vi "canDataSort.vi"() -> ()   [LabVIEW 2023]
panel:
  in  "canArrayDataIn":string[](array[string])
  in  "canArrayID_In":string[](array[string])
  in  "e":string="         2  1FFFFFFF   00000004    8        00\t00\tFF\tFF\tFF\tFF\tFF\tFF\r\n         3  0CF101A7   00000004    8        68\t00\t97\tCC\t00\t15\t39\t1A\r\n         2  1FFFFFFF   00000004    8        00\t00\tFF\tFF\tFF\tFF\tFF\tFF\r\n         3  0CF102A7   00000004    8        30\t75\tE0\t2E\t80\tFF\tFF\tFD\r\n         3  0CF101A7   00000004    8        68\t00\t97\tCC\t00\t15\t39\t1A\r\n         2  1FFFFFFF   00000004    8        00\t00\tFF\tFF\tFF\tFF\tFF\tFF\r\n        12  1FFFFFFF   00000004    8        00\t20\tFF\tFF\tFF\tFF\tFF\tFF\r\n         3  0CF102A7   00000004    8        30\t75\tE0\t2E\t80\tFF\tFF\tFD\r\n         3  0CF101A7   00000004    8        68\t00\t97\tCC\t00\t15\t39\t1A\r\n         2  1FFFFFFF   00000004    8        00\t00\tFF\tFF\tFF\tFF\tFF\tFF\r\n        22  1FFFFFFF   00000004    8        00\t20\tFF\tFF\tFF\tFF\tFF\tFF\r\n        12  1FFFFFFF   00000004    8        00\t20\tFF\tFF\tFF\tFF\tFF\tFF\r\n         3  0CF102A7   00000004    8        30\t75\tE0\t2E\t80\tFF\tFF\tFD\r\n         3  0CF101A7   00000004    8        68\t00\t97\tCC\t00\t15\t39\t1A\r\n         2  1FFFFFFF   00000004    8        00\t00\tFF\tFF\tFF\tFF\tFF\tFF\r\n        23  0CF101A7   00000004    8        68\t00\t97\tCC\t00\t15\t39\t1B\r\n        22  1FFFFFFF   00000004    8        00\t20\tFF\tFF\tFF\tFF\tFF\tFF\r\n        12  1FFFFFFF   00000004    8        00\t20\tFF\tFF\tFF\tFF\tFF\tFF\r\n         3  0CF102A7   00000004    8        30\t75\tE0\t2E\t80\tFF\tFF\tFD\r\n         3  0CF101A7   00000004    8        68\t00\t97\tCC\t00\t15\t39\t1A\r\n         2  1FFFFFFF   00000004    8        00\t00\tFF\tFF\tFF\tFF\tFF\tFF\r\n        23  0CF102A7   00000004    8        30\t75\tE0\t2E\t80\tFF\tFF\tFD\r\n        23  0CF101A7   00000004    8        68\t00\t97\tCC\t00\t15\t39\t1B\r\n        22  1FFFFFFF   00000004    8        00\t20\tFF\tFF\tFF\tFF\tFF\tFF\r\n        12  1FFFFFFF   00000004    8        00\t20\tFF\tFF\tFF\tFF\tFF\tFF\r\n         3  0CF102A7   00000004    8        30\t75\tE0\t2E\t80\tFF\tFF\tFD\r\n         3  0CF101A7   00000004    8        68\t00\t97\tCC\t00\t15\t39\t1A\r\n         2  1FFFFFFF   00000004    8        00\t00\tFF\tFF\tFF\tFF\tFF\tFF\r\n        32  1FFFFFFF   00000004    8        00\t20\tFF\tFF\tFF\tFF\tFF\tFF\r\n        23  0CF102A7   00000004    8        30\t75\tE0\t2E\t80\tFF\tFF\tFD\r\n        23  0CF101A7   00000004    8        68\t00\t97\tCC\t00\t15\t39\t1B\r\n        22  1FFFFFFF   00000004    8        00\t20\tFF\tFF\tFF\tFF\tFF\tFF\r\n        12  1FFFFFFF   00000004    8        00\t20\tFF\tFF\tFF\tFF\tFF\tFF\r\n         3  0CF102A7   00000004    8        30\t75\tE0\t2E\t80\tFF\tFF\tFD\r\n         3  0CF101A7   00000004    8        68\t00\t97\tCC\t00\t15\t39\t1A\r\n         2  1FFFFFFF   00000004    8        00\t00\tFF\tFF\tFF\tFF\tFF\tFF\r\n        41  18F11FF0   00000004    8        FF\t3F\t90\t68\t88\t1B\t10\t8C\r\n        32  1FFFFFFF   00000004    8        00\t20\tFF\tFF\tFF\tFF\tFF\tFF\r\n        23  0CF102A7   00000004    8        30\t75\tE0\t2E\t80\tFF\tFF\tFD\r\n        23  0CF101A7   00000004    8        68\t00\t97\tCC\t00\t15\t39\t1B\r\n        22  1FFFFFFF   00000004    8        00\t20\tFF\tFF\tFF\tFF\tFF\tFF\r\n        12  1FFFFFFF   00000004    8        00\t20\tFF\tFF\tFF\tFF\tFF\tFF\r\n         3  0CF102A7   00000004    8        30\t75\tE0\t2E\t80\tFF\tFF\tFD\r\n         3  0CF101A7   00000004    8        68\t00\t97\tCC\t00\t15\t39\t1A\r\n         2  1FFFFFFF   00000004    8        00\t00\tFF\tFF\tFF\tFF\tFF\tFF\r\n        42  18F120F0   00000004    8        2B\t75\t60\tB1\tB0\t01\tFF\tFF\r\n        41  18F11FF0   00000004    8        FF\t3F\t90\t68\t88\t1B\t10\t8C\r\n        32  1FFFFFFF   00000004    8        00\t20\tFF\tFF\tFF\tFF\tFF\tFF\r\n        23  0CF102A7   00000004    8        30\t75\tE0\t2E\t80\tFF\tFF\tFD\r\n        23  0CF101A7   00000004    8        68\t00\t97\tCC\t00\t15\t39\t1B\r\n        22  1FFFFFFF   00000004    8        00\t20\tFF\tFF\tFF\tFF\tFF\tFF\r\n        12  1FFFFFFF   00000004    8        00\t20\tFF\tFF\tFF\tFF\tFF\tFF\r\n         3  0CF102A7   00000004    8        30\t75\tE0\t2E\t80\tFF\tFF\tFD\r\n         3  0CF101A7   00000004    8        68\t00\t97\tCC\t00\t15\t39\t1A\r\n         2  1FFFFFFF   00000004    8        00\t00\tFF\tFF\tFF\tFF\tFF\tFF\r\n        43  0CF101A7   00000004    8        68\t00\t97\tCC\t00\t15\t39\t1C\r\n        42  18F120F0   00000004    8        2B\t75\t60\tB1\tB0\t01\tFF\tFF\r\n        41  18F11FF0   00000004    8        FF\t3F\t90\t68\t88\t1B\t10\t8C\r\n        32  1FFFFFFF   00000004    8        00\t20\tFF\tFF\tFF\tFF\tFF\tFF"
  in  "Boolean":bool
  out "canArrayData":string[](array[string])
  out "substring":string
  out "arrayIndex":i32
  out "whileIndex":i32
  out "index of element":i32
  out "canArrayID":string[](array[string])
  out "ID":string[](array[string])
  in  "b":string="      2043  0C3C4D4A   00000004    8        BE\tFF\tFF\t7F\t18\tFF\tFF\t4C\r\n      2043  0CF101A7   00000004    8        68\t00\t97\tCC\t00\t16\t39\t80\r\n      2042  18F120F0   00000004    8        2B\t75\t60\tB1\tB0\t01\tFF\tFF\r\n      2041  18F11FF0   00000004    8        FF\t3F\t90\t68\t88\t1B\t10\tCC\r\n      2032  1FFFFFFF   00000004    8        00\t00\tFF\tFF\tFF\tFF\tFF\tFF\r\n      2023  0CF102A7   00000004    8        30\t75\tE0\t2E\t80\tFF\tFF\tFD\r\n      2023  0CF101A7   00000004    8        68\t00\t97\tCC\t00\t16\t39\t7F\r\n      2022  1FFFFFFF   00000004    8        00\t00\tFF\tFF\tFF\tFF\tFF\tFF\r\n      2012  1FFFFFFF   00000004    8        00\t00\tFF\tFF\tFF\tFF\tFF\tFF\r\n      2003  0CF102A7   00000004    8        30\t75\tE0\t2E\t80\tFF\tFF\tFD\r\n      2044  0CF103A7   00000004    8        17\t1F\t08\t60\tB1\t1F\t08\t4C\r\n      2044  0CF102A7   00000004    8        30\t75\tE0\t2E\t80\tFF\tFF\tFD\r\n      2043  0C3C4D4A   00000004    8        BE\tFF\tFF\t7F\t18\tFF\tFF\t4C\r\n      2043  0CF101A7   00000004    8        68\t00\t97\tCC\t00\t16\t39\t80\r\n      2042  18F120F0   00000004    8        2B\t75\t60\tB1\tB0\t01\tFF\tFF\r\n      2041  18F11FF0   00000004    8        FF\t3F\t90\t68\t88\t1B\t10\tCC\r\n      2032  1FFFFFFF   00000004    8        00\t00\tFF\tFF\tFF\tFF\tFF\tFF\r\n      2023  0CF102A7   00000004    8        30\t75\tE0\t2E\t80\tFF\tFF\tFD\r\n      2023  0CF101A7   00000004    8        68\t00\t97\tCC\t00\t16\t39\t7F\r\n      2022  1FFFFFFF   00000004    8        00\t00\tFF\tFF\tFF\tFF\tFF\tFF\r\n      2012  1FFFFFFF   00000004    8        00\t00\tFF\tFF\tFF\tFF\tFF\tFF\r\n      2045  0CF104A7   00000004    8        F0\t60\t22\tFC\tFF\tFF\tFF\t4C\r\n      2044  0CF103A7   00000004    8        17\t1F\t08\t60\tB1\t1F\t08\t4C\r\n      2044  0CF102A7   00000004    8        30\t75\tE0\t2E\t80\tFF\tFF\tFD\r\n      2043  0C3C4D4A   00000004    8        BE\tFF\tFF\t7F\t18\tFF\tFF\t4C\r\n      2043  0CF101A7   00000004    8        68\t00\t97\tCC\t00\t16\t39\t80\r\n      2042  18F120F0   00000004    8        2B\t75\t60\tB1\tB0\t01\tFF\tFF\r\n      2041  18F11FF0   00000004    8        FF\t3F\t90\t68\t88\t1B\t10\tCC\r\n      2032  1FFFFFFF   00000004    8        00\t00\tFF\tFF\tFF\tFF\tFF\tFF\r\n      2023  0CF102A7   00000004    8        30\t75\tE0\t2E\t80\tFF\tFF\tFD\r\n      2023  0CF101A7   00000004    8        68\t00\t97\tCC\t00\t16\t39\t7F\r\n      2022  1FFFFFFF   00000004    8        00\t00\tFF\tFF\tFF\tFF\tFF\tFF\r\n      2045  18F106A7   00000004    8        00\tF7\tFF\tFF\tFF\tFF\tFF\t99\r\n      2045  0CF104A7   00000004    8        F0\t60\t22\tFC\tFF\tFF\tFF\t4C\r\n      2044  0CF103A7   00000004    8        17\t1F\t08\t60\tB1\t1F\t08\t4C\r\n      2044  0CF102A7   00000004    8        30\t75\tE0\t2E\t80\tFF\tFF\tFD\r\n      2043  0C3C4D4A   00000004    8        BE\tFF\tFF\t7F\t18\tFF\tFF\t4C\r\n      2043  0CF101A7   00000004    8        68\t00\t97\tCC\t00\t16\t39\t80\r\n      2042  18F120F0   00000004    8        2B\t75\t60\tB1\tB0\t01\tFF\tFF\r\n      2041  18F11FF0   00000004    8        FF\t3F\t90\t68\t88\t1B\t10\tCC\r\n      2032  1FFFFFFF   00000004    8        00\t00\tFF\tFF\tFF\tFF\tFF\tFF\r\n      2023  0CF102A7   00000004    8        30\t75\tE0\t2E\t80\tFF\tFF\tFD\r\n      2023  0CF101A7   00000004    8        68\t00\t97\tCC\t00\t16\t39\t7F\r\n      2046  18F121F0   00000004    8        09\t19\t00\t00\tFF\tFF\tB0\t01\r\n      2045  18F106A7   00000004    8        00\tF7\tFF\tFF\tFF\tFF\tFF\t99\r\n      2045  0CF104A7   00000004    8        F0\t60\t22\tFC\tFF\tFF\tFF\t4C\r\n      2044  0CF103A7   00000004    8        17\t1F\t08\t60\tB1\t1F\t08\t4C\r\n      2044  0CF102A7   00000004    8        30\t75\tE0\t2E\t80\tFF\tFF\tFD\r\n      2043  0C3C4D4A   00000004    8        BE\tFF\tFF\t7F\t18\tFF\tFF\t4C\r\n      2043  0CF101A7   00000004    8        68\t00\t97\tCC\t00\t16\t39\t80\r\n      2042  18F120F0   00000004    8        2B\t75\t60\tB1\tB0\t01\tFF\tFF\r\n      2041  18F11FF0   00000004    8        FF\t3F\t90\t68\t88\t1B\t10\tCC\r\n      2032  1FFFFFFF   00000004    8        00\t00\tFF\tFF\tFF\tFF\tFF\tFF\r\n      2023  0CF102A7   00000004    8        30\t75\tE0\t2E\t80\tFF\tFF\tFD\r\n      2047  1FFFFFFF   00000004    8        00\t00\tFF\tFF\tFF\tFF\tFF\tFF\r\n      2046  18F121F0   00000004    8        09\t19\t00\t00\tFF\tFF\tB0\t01\r\n      2045  18F106A7   00000004    8        00\tF7\tFF\tFF\tFF\tFF\tFF\t99\r\n      2045  0CF104A7   00000004    8        F0\t60\t22\tFC\tFF\tFF\tFF\t4C\r\n      2044  0CF103A7   00000004    8        17\t1F\t08\t60\tB1\t1F\t08\t4C\r\n      2044  0CF102A7   00000004    8        30\t75\tE0\t2E\t80\tFF\tFF\tFD\r\n      2043  0C3C4D4A   00000004    8        BE\tFF\tFF\t7F\t18\tFF\tFF\t4C\r\n      2043  0CF101A7   00000004    8        68\t00\t97\tCC\t00\t16\t39\t80\r\n      2042  18F120F0   00000004    8        2B\t75\t60\tB1\tB0\t01\tFF\tFF\r\n      2041  18F11FF0   00000004    8        FF\t3F\t90\t68\t88\t1B\t10\tCC\r\n      2032  1FFFFFFF   00000004    8        00\t00\tFF\tFF\tFF\tFF\tFF\tFF\r\n      2052  1FFFFFFF   00000004    8        00\t00\tFF\tFF\tFF\tFF\tFF\tFF\r\n      2047  1FFFFFFF   00000004    8        00\t00\tFF\tFF\tFF\tFF\tFF\tFF\r\n      2046  18F121F0   00000004    8        09\t19\t00\t00\tFF\tFF\tB0\t01\r\n      2045  18F106A7   00000004    8        00\tF7\tFF\tFF\tFF\tFF\tFF\t99\r\n      2045  0CF104A7   00000004    8        F0\t60\t22\tFC\tFF\tFF\tFF\t4C\r\n      2044  0CF103A7   00000004    8        17\t1F\t08\t60\tB1\t1F\t08\t4C\r\n      2044  0CF102A7   00000004    8        30\t75\tE0\t2E\t80\tFF\tFF\tFD\r\n      2043  0C3C4D4A   00000004    8        BE\tFF\tFF\t7F\t18\tFF\tFF\t4C\r\n      2043  0CF101A7   00000004    8        68\t00\t97\tCC\t00\t16\t39\t80\r\n      2042  18F120F0   00000004    8        2B\t75\t60\tB1\tB0\t01\tFF\tFF\r\n      2041  18F11FF0   00000004    8        FF\t3F\t90\t68\t88\t1B\t10\tCC\r\n      2062  1FFFFFFF   00000004    8        00\t00\tFF\tFF\tFF\tFF\tFF\tFF\r\n      2052  1FFFFFFF   00000004    8        00\t00\tFF\tFF\tFF\tFF\tFF\tFF\r\n      2047  1FFFFFFF   00000004    8        00\t00\tFF\tFF\tFF\tFF\tFF\tFF\r\n      2046  18F121F0   00000004    8        09\t19\t00\t00\tFF\tFF\tB0\t01\r\n      2045  18F106A7   00000004    8        00\tF7\tFF\tFF\tFF\tFF\tFF\t99\r\n      2045  0CF104A7   00000004    8        F0\t60\t22\tFC\tFF\tFF\tFF\t4C\r\n      2044  0CF103A7   00000004    8        17\t1F\t08\t60\tB1\t1F\t08\t4C\r\n      2044  0CF102A7   00000004    8        30\t75\tE0\t2E\t80\tFF\tFF\tFD"
  in  "c":string="      3712  1FFFFFFF   00000004    8        00\t20\tFF\tFF\tFF\tFF\tFF\tFF\r\n      3703  0CF102A7   00000004    8        30\t75\tE0\t2E\t80\tFF\tFF\tFD\r\n      3703  0CF101A7   00000004    8        68\t00\t97\tCC\t00\t19\t39\tD3\r\n      3702  1FFFFFFF   00000004    8        00\t20\tFF\tFF\tFF\tFF\tFF\tFF\r\n      3743  0C3C4D4A   00000004    8        BE\tFF\tFF\t7F\t18\tFF\tFF\t5D\r\n      3743  0CF101A7   00000004    8        68\t00\t97\tCC\t00\t19\t39\tD5\r\n      3742  18F120F0   00000004    8        2B\t75\t60\tB1\tB0\t01\tFF\tFF\r\n      3741  18F11FF0   00000004    8        FF\t3F\t90\t68\t88\t1B\t10\tDC\r\n      3732  1FFFFFFF   00000004    8        00\t20\tFF\tFF\tFF\tFF\tFF\tFF\r\n      3723  0CF102A7   00000004    8        30\t75\tE0\t2E\t80\tFF\tFF\tFD\r\n      3723  0CF101A7   00000004    8        68\t00\t97\tCC\t00\t19\t39\tD4\r\n      3722  1FFFFFFF   00000004    8        00\t20\tFF\tFF\tFF\tFF\tFF\tFF\r\n      3712  1FFFFFFF   00000004    8        00\t20\tFF\tFF\tFF\tFF\tFF\tFF\r\n      3703  0CF102A7   00000004    8        30\t75\tE0\t2E\t80\tFF\tFF\tFD\r\n      3703  0CF101A7   00000004    8        68\t00\t97\tCC\t00\t19\t39\tD3\r\n      3744  0CF102A7   00000004    8        30\t75\tE0\t2E\t80\tFF\tFF\tFD\r\n      3743  0C3C4D4A   00000004    8        BE\tFF\tFF\t7F\t18\tFF\tFF\t5D\r\n      3743  0CF101A7   00000004    8        68\t00\t97\tCC\t00\t19\t39\tD5\r\n      3742  18F120F0   00000004    8        2B\t75\t60\tB1\tB0\t01\tFF\tFF\r\n      3741  18F11FF0   00000004    8        FF\t3F\t90\t68\t88\t1B\t10\tDC\r\n      3732  1FFFFFFF   00000004    8        00\t20\tFF\tFF\tFF\tFF\tFF\tFF\r\n      3723  0CF102A7   00000004    8        30\t75\tE0\t2E\t80\tFF\tFF\tFD\r\n      3723  0CF101A7   00000004    8        68\t00\t97\tCC\t00\t19\t39\tD4\r\n      3722  1FFFFFFF   00000004    8        00\t20\tFF\tFF\tFF\tFF\tFF\tFF\r\n      3712  1FFFFFFF   00000004    8        00\t20\tFF\tFF\tFF\tFF\tFF\tFF\r\n      3703  0CF102A7   00000004    8        30\t75\tE0\t2E\t80\tFF\tFF\tFD\r\n      3744  0CF103A7   00000004    8        17\t1F\t08\t60\tB1\t1F\t08\t5D\r\n      3744  0CF102A7   00000004    8        30\t75\tE0\t2E\t80\tFF\tFF\tFD\r\n      3743  0C3C4D4A   00000004    8        BE\tFF\tFF\t7F\t18\tFF\tFF\t5D\r\n      3743  0CF101A7   00000004    8        68\t00\t97\tCC\t00\t19\t39\tD5\r\n      3742  18F120F0   00000004    8        2B\t75\t60\tB1\tB0\t01\tFF\tFF\r\n      3741  18F11FF0   00000004    8        FF\t3F\t90\t68\t88\t1B\t10\tDC\r\n      3732  1FFFFFFF   00000004    8        00\t20\tFF\tFF\tFF\tFF\tFF\tFF\r\n      3723  0CF102A7   00000004    8        30\t75\tE0\t2E\t80\tFF\tFF\tFD\r\n      3723  0CF101A7   00000004    8        68\t00\t97\tCC\t00\t19\t39\tD4\r\n      3722  1FFFFFFF   00000004    8        00\t20\tFF\tFF\tFF\tFF\tFF\tFF\r\n      3712  1FFFFFFF   00000004    8        00\t20\tFF\tFF\tFF\tFF\tFF\tFF\r\n      3745  0CF104A7   00000004    8        F0\t60\t22\tFC\tFF\tFF\tFF\t5D\r\n      3744  0CF103A7   00000004    8        17\t1F\t08\t60\tB1\t1F\t08\t5D\r\n      3744  0CF102A7   00000004    8        30\t75\tE0\t2E\t80\tFF\tFF\tFD\r\n      3743  0C3C4D4A   00000004    8        BE\tFF\tFF\t7F\t18\tFF\tFF\t5D\r\n      3743  0CF101A7   00000004    8        68\t00\t97\tCC\t00\t19\t39\tD5\r\n      3742  18F120F0   00000004    8        2B\t75\t60\tB1\tB0\t01\tFF\tFF\r\n      3741  18F11FF0   00000004    8        FF\t3F\t90\t68\t88\t1B\t10\tDC\r\n      3732  1FFFFFFF   00000004    8        00\t20\tFF\tFF\tFF\tFF\tFF\tFF\r\n      3723  0CF102A7   00000004    8        30\t75\tE0\t2E\t80\tFF\tFF\tFD\r\n      3723  0CF101A7   00000004    8        68\t00\t97\tCC\t00\t19\t39\tD4\r\n      3722  1FFFFFFF   00000004    8        00\t20\tFF\tFF\tFF\tFF\tFF\tFF\r\n      3745  18F106A7   00000004    8        00\tF7\tFF\tFF\tFF\tFF\tFF\tBB\r\n      3745  0CF104A7   00000004    8        F0\t60\t22\tFC\tFF\tFF\tFF\t5D\r\n      3744  0CF103A7   00000004    8        17\t1F\t08\t60\tB1\t1F\t08\t5D\r\n      3744  0CF102A7   00000004    8        30\t75\tE0\t2E\t80\tFF\tFF\tFD\r\n      3743  0C3C4D4A   00000004    8        BE\tFF\tFF\t7F\t18\tFF\tFF\t5D\r\n      3743  0CF101A7   00000004    8        68\t00\t97\tCC\t00\t19\t39\tD5"
  in  "d":string="      4683  0CF102A7   00000004    8        30\t75\tE0\t2E\t80\tFF\tFF\tFD\r\n      4683  0CF101A7   00000004    8        68\t00\t97\tCC\t00\t19\t39\t04\r\n      4682  1FFFFFFF   00000004    8        00\t20\tFF\tFF\tFF\tFF\tFF\tFF\r\n      4672  1FFFFFFF   00000004    8        00\t20\tFF\tFF\tFF\tFF\tFF\tFF\r\n      4663  0CF102A7   00000004    8        30\t75\tE0\t2E\t80\tFF\tFF\tFD\r\n      4662  0CF101A7   00000004    8        68\t00\t97\tCC\t00\t19\t39\t03\r\n      4662  1FFFFFFF   00000004    8        00\t20\tFF\tFF\tFF\tFF\tFF\tFF\r\n      4652  1FFFFFFF   00000004    8        00\t20\tFF\tFF\tFF\tFF\tFF\tFF\r\n      4702  0CF101A7   00000004    8        68\t00\t97\tCC\t00\t19\t39\t05\r\n      4702  1FFFFFFF   00000004    8        00\t20\tFF\tFF\tFF\tFF\tFF\tFF\r\n      4693  18F106A7   00000004    8        00\tF7\tFF\tFF\tFF\tFF\tFF\tCE\r\n      4692  1FFFFFFF   00000004    8        00\t00\tFF\tFF\tFF\tFF\tFF\tFF\r\n      4683  0CF102A7   00000004    8        30\t75\tE0\t2E\t80\tFF\tFF\tFD\r\n      4683  0CF101A7   00000004    8        68\t00\t97\tCC\t00\t19\t39\t04\r\n      4682  1FFFFFFF   00000004    8        00\t20\tFF\tFF\tFF\tFF\tFF\tFF\r\n      4672  1FFFFFFF   00000004    8        00\t20\tFF\tFF\tFF\tFF\tFF\tFF\r\n      4663  0CF102A7   00000004    8        30\t75\tE0\t2E\t80\tFF\tFF\tFD\r\n      4662  0CF101A7   00000004    8        68\t00\t97\tCC\t00\t19\t39\t03\r\n      4662  1FFFFFFF   00000004    8        00\t20\tFF\tFF\tFF\tFF\tFF\tFF\r\n"
  out "Array 3":string[](array[string])
  out "length 2":i32=1019337
  in  "a":string="         2  1FFFFFFF   00000004    8        00\t00\tFF\tFF\tFF\tFF\tFF\tFF\r\n         3  0CF101A7   00000004    8        68\t00\t97\tCC\t00\t15\t39\t1A\r\n         2  1FFFFFFF   00000004    8        00\t00\tFF\tFF\tFF\tFF\tFF\tFF\r\n         3  0CF102A7   00000004    8        30\t75\tE0\t2E\t80\tFF\tFF\tFD\r\n         3  0CF101A7   00000004    8        68\t00\t97\tCC\t00\t15\t39\t1A\r\n         2  1FFFFFFF   00000004    8        00\t00\tFF\tFF\tFF\tFF\tFF\tFF\r\n        12  1FFFFFFF   00000004    8        00\t20\tFF\tFF\tFF\tFF\tFF\tFF\r\n         3  0CF102A7   00000004    8        30\t75\tE0\t2E\t80\tFF\tFF\tFD\r\n         3  0CF101A7   00000004    8        68\t00\t97\tCC\t00\t15\t39\t1A\r\n         2  1FFFFFFF   00000004    8        00\t00\tFF\tFF\tFF\tFF\tFF\tFF\r\n        22  1FFFFFFF   00000004    8        00\t20\tFF\tFF\tFF\tFF\tFF\tFF\r\n        12  1FFFFFFF   00000004    8        00\t20\tFF\tFF\tFF\tFF\tFF\tFF\r\n         3  0CF102A7   00000004    8        30\t75\tE0\t2E\t80\tFF\tFF\tFD\r\n         3  0CF101A7   00000004    8        68\t00\t97\tCC\t00\t15\t39\t1A\r\n         2  1FFFFFFF   00000004    8        00\t00\tFF\tFF\tFF\tFF\tFF\tFF\r\n        23  0CF101A7   00000004    8        68\t00\t97\tCC\t00\t15\t39\t1B\r\n        22  1FFFFFFF   00000004    8        00\t20\tFF\tFF\tFF\tFF\tFF\tFF\r\n        12  1FFFFFFF   00000004    8        00\t20\tFF\tFF\tFF\tFF\tFF\tFF\r\n         3  0CF102A7   00000004    8        30\t75\tE0\t2E\t80\tFF\tFF\tFD\r\n         3  0CF101A7   00000004    8        68\t00\t97\tCC\t00\t15\t39\t1A\r\n         2  1FFFFFFF   00000004    8        00\t00\tFF\tFF\tFF\tFF\tFF\tFF\r\n        23  0CF102A7   00000004    8        30\t75\tE0\t2E\t80\tFF\tFF\tFD\r\n        23  0CF101A7   00000004    8        68\t00\t97\tCC\t00\t15\t39\t1B\r\n        22  1FFFFFFF   00000004    8        00\t20\tFF\tFF\tFF\tFF\tFF\tFF\r\n        12  1FFFFFFF   00000004    8        00\t20\tFF\tFF\tFF\tFF\tFF\tFF\r\n         3  0CF102A7   00000004    8        30\t75\tE0\t2E\t80\tFF\tFF\tFD\r\n         3  0CF101A7   00000004    8        68\t00\t97\tCC\t00\t15\t39\t1A\r\n         2  1FFFFFFF   00000004    8        00\t00\tFF\tFF\tFF\tFF\tFF\tFF\r\n        32  1FFFFFFF   00000004    8        00\t20\tFF\tFF\tFF\tFF\tFF\tFF\r\n        23  0CF102A7   00000004    8        30\t75\tE0\t2E\t80\tFF\tFF\tFD\r\n        23  0CF101A7   00000004    8        68\t00\t97\tCC\t00\t15\t39\t1B\r\n        22  1FFFFFFF   00000004    8        00\t20\tFF\tFF\tFF\tFF\tFF\tFF\r\n        12  1FFFFFFF   00000004    8        00\t20\tFF\tFF\tFF\tFF\tFF\tFF\r\n         3  0CF102A7   00000004    8        30\t75\tE0\t2E\t80\tFF\tFF\tFD\r\n         3  0CF101A7   00000004    8        68\t00\t97\tCC\t00\t15\t39\t1A\r\n         2  1FFFFFFF   00000004    8        00\t00\tFF\tFF\tFF\tFF\tFF\tFF\r\n        41  18F11FF0   00000004    8        FF\t3F\t90\t68\t88\t1B\t10\t8C\r\n        32  1FFFFFFF   00000004    8        00\t20\tFF\tFF\tFF\tFF\tFF\tFF\r\n        23  0CF102A7   00000004    8        30\t75\tE0\t2E\t80\tFF\tFF\tFD\r\n        23  0CF101A7   00000004    8        68\t00\t97\tCC\t00\t15\t39\t1B\r\n        22  1FFFFFFF   00000004    8        00\t20\tFF\tFF\tFF\tFF\tFF\tFF\r\n        12  1FFFFFFF   00000004    8        00\t20\tFF\tFF\tFF\tFF\tFF\tFF\r\n         3  0CF102A7   00000004    8        30\t75\tE0\t2E\t80\tFF\tFF\tFD\r\n         3  0CF101A7   00000004    8        68\t00\t97\tCC\t00\t15\t39\t1A\r\n         2  1FFFFFFF   00000004    8        00\t00\tFF\tFF\tFF\tFF\tFF\tFF\r\n        42  18F120F0   00000004    8        2B\t75\t60\tB1\tB0\t01\tFF\tFF\r\n        41  18F11FF0   00000004    8        FF\t3F\t90\t68\t88\t1B\t10\t8C\r\n        32  1FFFFFFF   00000004    8        00\t20\tFF\tFF\tFF\tFF\tFF\tFF\r\n        23  0CF102A7   00000004    8        30\t75\tE0\t2E\t80\tFF\tFF\tFD\r\n        23  0CF101A7   00000004    8        68\t00\t97\tCC\t00\t15\t39\t1B\r\n        22  1FFFFFFF   00000004    8        00\t20\tFF\tFF\tFF\tFF\tFF\tFF\r\n        12  1FFFFFFF   00000004    8        00\t20\tFF\tFF\tFF\tFF\tFF\tFF\r\n         3  0CF102A7   00000004    8        30\t75\tE0\t2E\t80\tFF\tFF\tFD\r\n         3  0CF101A7   00000004    8        68\t00\t97\tCC\t00\t15\t39\t1A\r\n         2  1FFFFFFF   00000004    8        00\t00\tFF\tFF\tFF\tFF\tFF\tFF\r\n        43  0CF101A7   00000004    8        68\t00\t97\tCC\t00\t15\t39\t1C\r\n        42  18F120F0   00000004    8        2B\t75\t60\tB1\tB0\t01\tFF\tFF\r\n        41  18F11FF0   00000004    8        FF\t3F\t90\t68\t88\t1B\t10\t8C\r\n        32  1FFFFFFF   00000004    8        00\t20\tFF\tFF\tFF\tFF\tFF\tFF"
  in  "raw":string="         2  1FFFFFFF   00000004    8        00\t00\tFF\tFF\tFF\tFF\tFF\tFF\r\n         3  0CF101A7   00000004    8        68\t00\t97\tCC\t00\t15\t39\t1A\r\n         2  1FFFFFFF   00000004    8        00\t00\tFF\tFF\tFF\tFF\tFF\tFF\r\n         3  0CF102A7   00000004    8        30\t75\tE0\t2E\t80\tFF\tFF\tFD\r\n         3  0CF101A7   00000004    8        68\t00\t97\tCC\t00\t15\t39\t1A\r\n         2  1FFFFFFF   00000004    8        00\t00\tFF\tFF\tFF\tFF\tFF\tFF\r\n        12  1FFFFFFF   00000004    8        00\t20\tFF\tFF\tFF\tFF\tFF\tFF\r\n         3  0CF102A7   00000004    8        30\t75\tE0\t2E\t80\tFF\tFF\tFD\r\n         3  0CF101A7   00000004    8        68\t00\t97\tCC\t00\t15\t39\t1A\r\n         2  1FFFFFFF   00000004    8        00\t00\tFF\tFF\tFF\tFF\tFF\tFF\r\n        22  1FFFFFFF   00000004    8        00\t20\tFF\tFF\tFF\tFF\tFF\tFF\r\n        12  1FFFFFFF   00000004    8        00\t20\tFF\tFF\tFF\tFF\tFF\tFF\r\n         3  0CF102A7   00000004    8        30\t75\tE0\t2E\t80\tFF\tFF\tFD\r\n         3  0CF101A7   00000004    8        68\t00\t97\tCC\t00\t15\t39\t1A\r\n         2  1FFFFFFF   00000004    8        00\t00\tFF\tFF\tFF\tFF\tFF\tFF\r\n        23  0CF101A7   00000004    8        68\t00\t97\tCC\t00\t15\t39\t1B\r\n        22  1FFFFFFF   00000004    8        00\t20\tFF\tFF\tFF\tFF\tFF\tFF\r\n        12  1FFFFFFF   00000004    8        00\t20\tFF\tFF\tFF\tFF\tFF\tFF\r\n         3  0CF102A7   00000004    8        30\t75\tE0\t2E\t80\tFF\tFF\tFD\r\n         3  0CF101A7   00000004    8        68\t00\t97\tCC\t00\t15\t39\t1A\r\n         2  1FFFFFFF   00000004    8        00\t00\tFF\tFF\tFF\tFF\tFF\tFF\r\n        23  0CF102A7   00000004    8        30\t75\tE0\t2E\t80\tFF\tFF\tFD\r\n        23  0CF101A7   00000004    8        68\t00\t97\tCC\t00\t15\t39\t1B\r\n        22  1FFFFFFF   00000004    8        00\t20\tFF\tFF\tFF\tFF\tFF\tFF\r\n        12  1FFFFFFF   00000004    8        00\t20\tFF\tFF\tFF\tFF\tFF\tFF\r\n         3  0CF102A7   00000004    8        30\t75\tE0\t2E\t80\tFF\tFF\tFD\r\n         3  0CF101A7   00000004    8        68\t00\t97\tCC\t00\t15\t39\t1A\r\n         2  1FFFFFFF   00000004    8        00\t00\tFF\tFF\tFF\tFF\tFF\tFF\r\n        32  1FFFFFFF   00000004    8        00\t20\tFF\tFF\tFF\tFF\tFF\tFF\r\n        23  0CF102A7   00000004    8        30\t75\tE0\t2E\t80\tFF\tFF\tFD\r\n        23  0CF101A7   00000004    8        68\t00\t97\tCC\t00\t15\t39\t1B\r\n        22  1FFFFFFF   00000004    8        00\t20\tFF\tFF\tFF\tFF\tFF\tFF\r\n        12  1FFFFFFF   00000004    8        00\t20\tFF\tFF\tFF\tFF\tFF\tFF\r\n         3  0CF102A7   00000004    8        30\t75\tE0\t2E\t80\tFF\tFF\tFD\r\n         3  0CF101A7   00000004    8        68\t00\t97\tCC\t00\t15\t39\t1A\r\n         2  1FFFFFFF   00000004    8        00\t00\tFF\tFF\tFF\tFF\tFF\tFF\r\n        41  18F11FF0   00000004    8        FF\t3F\t90\t68\t88\t1B\t10\t8C\r\n        32  1FFFFFFF   00000004    8        00\t20\tFF\tFF\tFF\tFF\tFF\tFF\r\n        23  0CF102A7   00000004    8        30\t75\tE0\t2E\t80\tFF\tFF\tFD\r\n        23  0CF101A7   00000004    8        68\t00\t97\tCC\t00\t15\t39\t1B\r\n        22  1FFFFFFF   00000004    8        00\t20\tFF\tFF\tFF\tFF\tFF\tFF\r\n        12  1FFFFFFF   00000004    8        00\t20\tFF\tFF\tFF\tFF\tFF\tFF\r\n         3  0CF102A7   00000004    8        30\t75\tE0\t2E\t80\tFF\tFF\tFD\r\n         3  0CF101A7   00000004    8        68\t00\t97\tCC\t00\t15\t39\t1A\r\n         2  1FFFFFFF   00000004    8        00\t00\tFF\tFF\tFF\tFF\tFF\tFF\r\n        42  18F120F0   00000004    8        2B\t75\t60\tB1\tB0\t01\tFF\tFF\r\n        41  18F11FF0   00000004    8        FF\t3F\t90\t68\t88\t1B\t10\t8C\r\n        32  1FFFFFFF   00000004    8        00\t20\tFF\tFF\tFF\tFF\tFF\tFF\r\n        23  0CF102A7   00000004    8        30\t75\tE0\t2E\t80\tFF\tFF\tFD\r\n        23  0CF101A7   00000004    8        68\t00\t97\tCC\t00\t15\t39\t1B\r\n        22  1FFFFFFF   00000004    8        00\t20\tFF\tFF\tFF\tFF\tFF\tFF\r\n        12  1FFFFFFF   00000004    8        00\t20\tFF\tFF\tFF\tFF\tFF\tFF\r\n         3  0CF102A7   00000004    8        30\t75\tE0\t2E\t80\tFF\tFF\tFD\r\n         3  0CF101A7   00000004    8        68\t00\t97\tCC\t00\t15\t39\t1A\r\n         2  1FFFFFFF   00000004    8        00\t00\tFF\tFF\tFF\tFF\tFF\tFF\r\n        43  0CF101A7   00000004    8        68\t00\t97\tCC\t00\t15\t39\t1C\r\n        42  18F120F0   00000004    8        2B\t75\t60\tB1\tB0\t01\tFF\tFF\r\n        41  18F11FF0   00000004    8        FF\t3F\t90\t68\t88\t1B\t10\t8C\r\n        32  1FFFFFFF   00000004    8        00\t20\tFF\tFF\tFF\tFF\tFF\tFF\r\n        23  0CF102A7   00000004    8        30\t75\tE0\t2E\t80\tFF\tFF\tFD\r\n        23  0CF101A7   00000004    8        68\t00\t97\tCC\t00\t15\t39\t1B\r\n        22  1FFFFFFF   00000004    8        00\t20\tFF\tFF\tFF\tFF\tFF\tFF\r\n        12  1FFFFFFF   00000004    8        00\t20\tFF\tFF\tFF\tFF\tFF\tFF\r\n         3  0CF102A7   00000004    8        30\t75\tE0\t2E\t80\tFF\tFF\tFD\r\n         3  0CF101A7   00000004    8        68\t00\t97\tCC\t00\t15\t39\t1A\r\n         2  1FFFFFFF   00000004    8        00\t00\tFF\tFF\tFF\tFF\tFF\tFF\r\n        43  0C3C4D4A   00000004    8        BE\tFF\tFF\t7F\t18\tFF\tFF\t38\r\n        43  0CF101A7   00000004    8        68\t00\t97\tCC\t00\t15\t39\t1C\r\n        42  18F120F0   00000004    8        2B\t75\t60\tB1\tB0\t01\tFF\tFF\r\n        41  18F11FF0   00000004    8        FF\t3F\t90\t68\t88\t1B\t10\t8C\r\n        32  1FFFFFFF   00000004    8        00\t20\tFF\tFF\tFF\tFF\tFF\tFF\r\n        23  0CF102A7   00000004    8        30\t75\tE0\t2E\t80\tFF\tFF\tFD\r\n        23  0CF101A7   00000004    8        68\t00\t97\tCC\t00\t15\t39\t1B\r\n        22  1FFFFFFF   00000004    8        00\t20\tFF\tFF\tFF\tFF\tFF\tFF\r\n        12  1FFFFFFF   00000004    8        00\t20\tFF\tFF\tFF\tFF\tFF\tFF\r\n         3  0CF102A7   00000004    8        30\t75\tE0\t2E\t80\tFF\tFF\tFD\r\n         3  0CF101A7   00000004    8        68\t00\t97\tCC\t00\t15\t39\t1A\r\n        44  0CF102A7   00000004    8        30\t75\tE0\t2E\t80\tFF\tFF\tFD\r\n        43  0C3C4D4A   00000004    8        BE\tFF\tFF\t7F\t18\tFF\tFF\t38\r\n        43  0CF101A7   00000004    8        68\t00\t97\tCC\t00\t15\t39\t1C\r\n        42  18F120F0   00000004    8        2B\t75\t60\tB1\tB0\t01\tFF\tFF\r\n        41  18F11FF0   00000004    8        FF\t3F\t90\t68\t88\t1B\t10\t8C\r\n        32  1FFFFFFF   00000004    8        00\t20\tFF\tFF\tFF\tFF\tFF\tFF\r\n        23  0CF102A7   00000004    8        30\t75\tE0\t2E\t80\tFF\tFF\tFD\r\n        23  0CF101A7   00000004    8        68\t00\t97\tCC\t00\t15\t39\t1B\r\n        22  1FFFFFFF   00000004    8        00\t20\tFF\tFF\tFF\tFF\tFF\tFF\r\n        12  1FFFFFFF   00000004    8        00\t20\tFF\tFF\tFF\tFF\tFF\tFF\r\n         3  0CF102A7   00000004    8        30\t75\tE0\t2E\t80\tFF\tFF\tFD\r\n        44  0CF103A7   00000004    8        17\t1F\t08\t60\tB1\t1F\t08\t38\r\n        44  0CF102A7   00000004    8        30\t75\tE0\t2E\t80\tFF\tFF\tFD\r\n        43  0C3C4D4A   00000004    8        BE\tFF\tFF\t7F\t18\tFF\tFF\t38\r\n        43  0CF101A7   00000004    8        68\t00\t97\tCC\t00\t15\t39\t1C\r\n        42  18F120F0   00000004    8        2B\t75\t60\tB1\tB0\t01\tFF\tFF\r\n        41  18F11FF0   00000004    8        FF\t3F\t90\t68\t88\t1B\t10\t8C\r\n        32  1FFFFFFF   00000004    8        00\t20\tFF\tFF\tFF\tFF\tFF\tFF\r\n        23  0CF102A7   00000004    8        30\t75\tE0\t2E\t80\tFF\tFF\tFD\r\n        23  0CF101A7   00000004    8        68\t00\t97\tCC\t00\t15\t39\t1B\r\n        22  1FFFFFFF   00000004    8        00\t20\tFF\tFF\tFF\tFF\tFF\tFF\r\n        12  1FFFFFFF   00000004    8        00\t20\tFF\tFF\tFF\tFF\tFF\tFF\r\n        45  0CF104A7   00000004    8        F0\t60\t22\tFC\tFF\tFF\tFF\t38\r\n        44  0CF103A7   00000004    8        17\t1F\t08\t60\tB1\t1F\t08\t38\r\n        44  0CF102A7   00000004    8        30\t75\tE0\t2E\t80\tFF\tFF\tFD\r\n        43  0C3C4D4A   00000004    8        BE\tFF\tFF\t7F\t18\tFF\tFF\t38\r\n        43  0CF101A7   00000004    8        68\t00\t97\tCC\t00\t15\t39\t1C\r\n        42  18F120F0   00000004    8        2B\t75\t60\tB1\tB0\t01\tFF\tFF\r\n        41  18F11FF0   00000004    8        FF\t3F\t90\t68\t88\t1B\t10\t8C\r\n        32  1FFFFFFF   00000004    8        00\t20\tFF\tFF\tFF\tFF\tFF\tFF\r\n        23  0CF102A7   00000004    8        30\t75\tE0\t2E\t80\tFF\tFF\tFD\r\n        23  0CF101A7   00000004    8        68\t00\t97\tCC\t00\t15\t39\t1B\r\n        22  1FFFFFFF   00000004    8        00\t20\tFF\tFF\tFF\tFF\tFF\tFF\r\n        46  18F106A7   00000004    8        00\tF7\tFF\tFF\tFF\tFF\tFF\t71\r\n        45  0CF104A7   00000004    8        F0\t60\t22\tFC\tFF\tFF\tFF\t38\r\n        44  0CF103A7   00000004    8        17\t1F\t08\t60\tB1\t1F\t08\t38\r\n        44  0CF102A7   00000004    8        30\t75\tE0\t2E\t80\tFF\tFF\tFD\r\n        43  0C3C4D4A   00000004    8        BE\tFF\tFF\t7F\t18\tFF\tFF\t38\r\n        43  0CF101A7   00000004    8        68\t00\t97\tCC\t00\t15\t39\t1C\r\n        42  18F120F0   00000004    8        2B\t75\t60\tB1\tB0\t01\tFF\tFF\r\n        41  18F11FF0   00000004    8        FF\t3F\t90\t68\t88\t1B\t10\t8C\r\n        32  1FFFFFFF   00000004    8        00\t20\tFF\tFF\tFF\tFF\tFF\tFF\r\n        23  0CF102A7   00000004    8        30\t75\tE0\t2E\t80\tFF\tFF\tFD\r\n        23  0CF101A7   00000004    8        68\t00\t97\tCC\t00\t15\t39\t1B\r\n        46  18F121F0   00000004    8        09\t16\t00\t00\tFF\tFF\tB0\t01\r\n        46  18F106A7   00000004    8        00\tF7\tFF\tFF\tFF\tFF\tFF\t71\r\n        45  0CF104A7   00000004    8        F0\t60\t22\tFC\tFF\tFF\tFF\t38\r\n        44  0CF103A7   00000004    8        17\t1F\t08\t60\tB1\t1F\t08\t38\r\n        44  0CF102A7   00000004    8        30\t75\tE0\t2E\t80\tFF\tFF\tFD\r\n        43  0C3C4D4A   00000004    8        BE\tFF\tFF\t7F\t18\tFF\tFF\t38\r\n        43  0CF101A7   00000004    8        68\t00\t97\tCC\t00\t15\t39\t1C\r\n        42  18F120F0   00000004    8        2B\t75\t60\tB1\tB0\t01\tFF\tFF\r\n        41  18F11FF0   00000004    8        FF\t3F\t90\t68\t88\t1B\t10\t8C\r\n        32  1FFFFFFF   00000004    8        00\t20\tFF\tFF\tFF\tFF\tFF\tFF\r\n        23  0CF102A7   00000004    8        30\t75\tE0\t2E\t80\tFF\tFF\tFD\r\n        47  1FFFFFFF   00000004    8        00\t00\tFF\tFF\tFF\tFF\tFF\tFF\r\n        46  18F121F0   00000004    8        09\t16\t00\t00\tFF\tFF\tB0\t01\r\n        46  18F106A7   00000004    8        00\tF7\tFF\tFF\tFF\tFF\tFF\t71\r\n        45  0CF104A7   00000004    8        F0\t60\t22\tFC\tFF\tFF\tFF\t38\r\n        44  0CF103A7   00000004    8        17\t1F\t08\t60\tB1\t1F\t08\t38\r\n        44  0CF102A7   00000004    8        30\t75\tE0\t2E\t80\tFF\tFF\tFD\r\n        43  0C3C4D4A   00000004    8        BE\tFF\tFF\t7F\t18\tFF\tFF\t38\r\n        43  0CF101A7   00000004    8        68\t00\t97\tCC\t00\t15\t39\t1C\r\n        42  18F120F0   00000004    8        2B\t75\t60\tB1\tB0\t01\tFF\tFF\r\n        41  18F11FF0   00000004    8        FF\t3F\t90\t68\t88\t1B\t10\t8C\r\n        32  1FFFFFFF   00000004    8        00\t20\tFF\tFF\tFF\tFF\tFF\tFF\r\n        52  1FFFFFFF   00000004    8        00\t00\tFF\tFF\tFF\tFF\tFF\tFF\r\n        47  1FFFFFFF   00000004    8        00\t00\tFF\tFF\tFF\tFF\tFF\tFF\r\n        46  18F121F0   00000004    8        09\t16\t00\t00\tFF\tFF\tB0\t01\r\n        46  18F106A7   00000004    8        00\tF7\tFF\tFF\tFF\tFF\tFF\t71\r\n        45  0CF104A7   00000004    8        F0\t60\t22\tFC\tFF\tFF\tFF\t38\r\n        44  0CF103A7   00000004    8        17\t1F\t08\t60\tB1\t1F\t08\t38\r\n        44  0CF102A7   00000004    8        30\t75\tE0\t2E\t80\tFF\tFF\tFD\r\n        43  0C3C4D4A   00000004    8        BE\tFF\tFF\t7F\t18\tFF\tFF\t38\r\n        43  0CF101A7   00000004    8        68\t00\t97\tCC\t00\t15\t39\t1C\r\n        42  18F120F0   00000004    8        2B\t75\t60\tB1\tB0\t01\tFF\tFF\r\n        41  18F11FF0   00000004    8        FF\t3F\t90\t68\t88\t1B\t10\t8C\r\n        62  1FFFFFFF   00000004    8        00\t20\tFF\tFF\tFF\tFF\tFF\tFF\r\n        52  1FFFFFFF   00000004    8        00\t00\tFF\tFF\tFF\tFF\tFF\tFF\r\n        47  1FFFFFFF   00000004    8        00\t00\tFF\tFF\tFF\tFF\tFF\tFF\r\n        46  18F121F0   00000004    8        09\t16\t00\t00\tFF\tFF\tB0\t01\r\n        46  18F106A7   00000004    8        00\tF7\tFF\tFF\tFF\tFF\tFF\t71\r\n        45  0CF104A7   00000004    8        F0\t60\t22\tFC\tFF\tFF\tFF\t38\r\n        44  0CF103A7   00000004    8        17\t1F\t08\t60\tB1\t1F\t08\t38\r\n        44  0CF102A7   00000004    8        30\t75\tE0\t2E\t80\tFF\tFF\tFD\r\n        43  0C3C4D4A   00000004    8        BE\tFF\tFF\t7F\t18\tFF\tFF\t38\r\n        43  0CF101A7   00000004    8        68\t00\t97\tCC\t00\t15\t39\t1C\r\n        42  18F120F0   00000004    8        2B\t75\t60\tB1\tB0\t01\tFF\tFF\r\n        63  0CF101A7   00000004    8        68\t00\t97\tCC\t00\t15\t39\t1D\r\n        62  1FFFFFFF   00000004    8        00\t20\tFF\tFF\tFF\tFF\tFF\tFF\r\n        52  1FFFFFFF   00000004    8        00\t00\tFF\tFF\tFF\tFF\tFF\tFF\r\n        47  1FFFFFFF   00000004    8        00\t00\tFF\tFF\tFF\tFF\tFF\tFF\r\n        46  18F121F0   00000004    8        09\t16\t00\t00\tFF\tFF\tB0\t01\r\n        46  18F106A7   00000004    8        00\tF7\tFF\tFF\tFF\tFF\tFF\t71\r\n        45  0CF104A7   00000004    8        F0\t60\t22\tFC\tFF\tFF\tFF\t38\r\n        44  0CF103A7   00000004    8        17\t1F\t08\t60\tB1\t1F\t08\t38\r\n        44  0CF102A7   00000004    8        30\t75\tE0\t2E\t80\tFF\tFF\tFD\r\n        43  0C3C4D4A   00000004    8        BE\tFF\tFF\t7F\t18\tFF\tFF\t38\r\n        43  0CF101A7   00000004    8        68\t00\t97\tCC\t00\t15\t39\t1C\r\n        63  0CF102A7   00000004    8        30\t75\tE0\t2E\t80\tFF\tFF\tFD\r\n        63  0CF101A7   00000004    8        68\t00\t97\tCC\t00\t15\t39\t1D\r\n        62  1FFFFFFF   00000004    8        00\t20\tFF\tFF\tFF\tFF\tFF\tFF\r\n        52  1FFFFFFF   00000004    8        00\t00\tFF\tFF\tFF\tFF\tFF\tFF\r\n        47  1FFFFFFF   00000004    8        00\t00\tFF\tFF\tFF\tFF\tFF\tFF\r\n        46  18F121F0   00000004    8        09\t16\t00\t00\tFF\tFF\tB0\t01\r\n        46  18F106A7   00000004    8        00\tF7\tFF\tFF\tFF\tFF\tFF\t71\r\n        45  0CF104A7   00000004    8        F0\t60\t22\tFC\tFF\tFF\tFF\t38\r\n        44  0CF103A7   00000004    8        17\t1F\t08\t60\tB1\t1F\t08\t38\r\n        44  0CF102A7   00000004    8        30\t75\tE0\t2E\t80\tFF\tFF\tFD\r\n        43  0C3C4D4A   00000004    8        BE\tFF\tFF\t7F\t18\tFF\tFF\t38\r\n        72  1FFFFFFF   00000004    8        00\t00\tFF\tFF\tFF\tFF\tFF\tFF\r\n        63  0CF102A7   00000004    8        30\t75\tE0\t2E\t80\tFF\tFF\tFD\r\n        63  0CF101A7   00000004    8        68\t00\t97\tCC\t00\t15\t39\t1D\r\n        62  1FFFFFFF   00000004    8        00\t20\tFF\tFF\tFF\tFF\tFF\tFF\r\n        52  1FFFFFFF   00000004    8        00\t00\tFF\tFF\tFF\tFF\tFF\tFF\r\n        47  1FFFFFFF   00000004    8        00\t00\tFF\tFF\tFF\tFF\tFF\tFF\r\n        46  18F121F0   00000004    8        09\t16\t00\t00\tFF\tFF\tB0\t01\r\n        46  18F106A7   00000004    8        00\tF7\tFF\tFF\tFF\tFF\tFF\t71\r\n        45  0CF104A7   00000004    8        F0\t60\t22\tFC\tFF\tFF\tFF\t38\r\n        44  0CF103A7   00000004    8        17\t1F\t08\t60\tB1\t1F\t08\t38\r\n        44  0CF102A7   00000004    8        30\t75\tE0\t2E\t80\tFF\tFF\tFD\r\n        82  1FFFFFFF   00000004    8        00\t20\tFF\tFF\tFF\tFF\tFF\tFF\r\n        72  1FFFFFFF   00000004    8        00\t00\tFF\tFF\tFF\tFF\tFF\tFF\r\n        63  0CF102A7   00000004    8        30\t75\tE0\t2E\t80\tFF\tFF\tFD\r\n        63  0CF101A7   00000004    8        68\t00\t97\tCC\t00\t15\t39\t1D\r\n        62  1FFFFFFF   00000004    8        00\t20\tFF\tFF\tFF\tFF\tFF\tFF\r\n        52  1FFFFFFF   00000004    8        00\t00\tFF\tFF\tFF\tFF\tFF\tFF\r\n        47  1FFFFFFF   00000004    8        00\t00\tFF\tFF\tFF\tFF\tFF\tFF\r\n        46  18F121F0   00000004    8        09\t16\t00\t00\tFF\tFF\tB0\t01\r\n        46  18F106A7   00000004    8        00\tF7\tFF\tFF\tFF\tFF\tFF\t71\r\n        45  0CF104A7   00000004    8        F0\t60\t22\tFC\tFF\tFF\tFF\t38\r\n        44  0CF103A7   00000004    8        17\t1F\t08\t60\tB1\t1F\t08\t38\r\n        83  0CF101A7   00000004    8        68\t00\t97\tCC\t00\t15\t39\t1E\r\n        82  1FFFFFFF   00000004    8        00\t20\tFF\tFF\tFF\tFF\tFF\tFF\r\n        72  1FFFFFFF   00000004    8        00\t00\tFF\tFF\tFF\tFF\tFF\tFF\r\n        63  0CF102A7   00000004    8        30\t75\tE0\t2E\t80\tFF\tFF\tFD\r\n        63  0CF101A7   00000004    8        68\t00\t97\tCC\t00\t15\t39\t1D\r\n        62  1FFFFFFF   00000004    8        00\t20\tFF\tFF\tFF\tFF\tFF\tFF\r\n        52  1FFFFFFF   00000004    8        00\t00\tFF\tFF\tFF\tFF\tFF\tFF\r\n        47  1FFFFFFF   00000004    8        00\t00\tFF\tFF\tFF\tFF\tFF\tFF\r\n        46  18F121F0   00000004    8        09\t16\t00\t00\tFF\tFF\tB0\t01\r\n        46  18F106A7   00000004    8        00\tF7\tFF\tFF\tFF\tFF\tFF\t71\r\n        45  0CF104A7   00000004    8        F0\t60\t22\tFC\tFF\tFF\tFF\t38\r\n        83  0CF102A7   00000004    8        30\t75\tE0\t2E\t80\tFF\tFF\tFD\r\n        83  0CF101A7   00000004    8        68\t00\t97\tCC\t00\t15\t39\t1E\r\n        82  1FFFFFFF   00000004    8        00\t20\tFF\tFF\tFF\tFF\tFF\tFF\r\n        72  1FFFFFFF   00000004    8        00\t00\tFF\tFF\tFF\tFF\tFF\tFF\r\n        63  0CF102A7   00000004    8        30\t75\tE0\t2E\t80\tFF\tFF\tFD\r\n        63  0CF101A7   00000004    8        68\t00\t97\tCC\t00\t15\t39\t1D\r\n        62  1FFFFFFF   00000004    8        00\t20\tFF\tFF\tFF\tFF\tFF\tFF\r\n        52  1FFFFFFF   00000004    8        00\t00\tFF\tFF\tFF\tFF\tFF\tFF\r\n        47  1FFFFFFF   00000004    8        00\t00\tFF\tFF\tFF\tFF\tFF\tFF\r\n        46  18F121F0   00000004    8        09\t16\t00\t00\tFF\tFF\tB0\t01\r\n        46  18F106A7   00000004    8        00\tF7\tFF\tFF\tFF\tFF\tFF\t71\r\n        92  1FFFFFFF   00000004    8        00\t00\tFF\tFF\tFF\tFF\tFF\tFF\r\n        83  0CF102A7   00000004    8        30\t75\tE0\t2E\t80\tFF\tFF\tFD\r\n        83  0CF101A7   00000004    8        68\t00\t97\tCC\t00\t15\t39\t1E\r\n        82  1FFFFFFF   00000004    8        00\t20\tFF\tFF\tFF\tFF\tFF\tFF\r\n        72  1FFFFFFF   00000004    8        00\t00\tFF\tFF\tFF\tFF\tFF\tFF\r\n        63  0CF102A7   00000004    8        30\t75\tE0\t2E\t80\tFF\tFF\tFD\r\n        63  0CF101A7   00000004    8        68\t00\t97\tCC\t00\t15\t39\t1D\r\n        62  1FFFFFFF   00000004    8        00\t20\tFF\tFF\tFF\tFF\tFF\tFF\r\n        52  1FFFFFFF   00000004    8        00\t00\tFF\tFF\tFF\tFF\tFF\tFF\r\n        47  1FFFFFFF   00000004    8        00\t00\tFF\tFF\tFF\tFF\tFF\tFF\r\n        46  18F121F0   00000004    8        09\t16\t00\t00\tFF\tFF\tB0\t01\r\n        93  18F106A7   00000004    8        00\tF7\tFF\tFF\tFF\tFF\tFF\t72\r\n        92  1FFFFFFF   00000004    8        00\t00\tFF\tFF\tFF\tFF\tFF\tFF\r\n        83  0CF102A7   00000004    8        30\t75\tE0\t2E\t80\tFF\tFF\tFD\r\n        83  0CF101A7   00000004    8        68\t00\t97\tCC\t00\t15\t39\t1E\r\n        82  1FFFFFFF   00000004    8        00\t20\tFF\tFF\tFF\tFF\tFF\tFF\r\n        72  1FFFFFFF   00000004    8        00\t00\tFF\tFF\tFF\tFF\tFF\tFF\r\n        63  0CF102A7   00000004    8        30\t75\tE0\t2E\t80\tFF\tFF\tFD\r\n        63  0CF101A7   00000004    8        68\t00\t97\tCC\t00\t15\t39\t1D\r\n        62  1FFFFFFF   00000004    8        00\t20\tFF\tFF\tFF\tFF\tFF\tFF\r\n        52  1FFFFFFF   00000004    8        00\t00\tFF\tFF\tFF\tFF\tFF\tFF\r\n        47  1FFFFFFF   00000004    8        00\t00\tFF\tFF\tFF\tFF\tFF\tFF\r\n       102  1FFFFFFF   00000004    8        00\t20\tFF\tFF\tFF\tFF\tFF\tFF\r\n        93  18F106A7   00000004    8        00\tF7\tFF\tFF\tFF\tFF\tFF\t72\r\n        92  1FFFFFFF   00000004    8        00\t00\tFF\tFF\tFF\tFF\tFF\tFF\r\n        83  
